vi "Window Title.vi"(0 "LV RT in":refnum<class "LV RT.lvclass">, 5 "VI Reference":refnum<vi>, 11 "error in (no error)":errorcluster) -> (4 "LV RT out":refnum<class "LV RT.lvclass">, 6 "Window Title":string, 15 "error out":errorcluster)   [LabVIEW 2016, in "LV RT.lvclass"]
uses:
  LV RT.lvclass
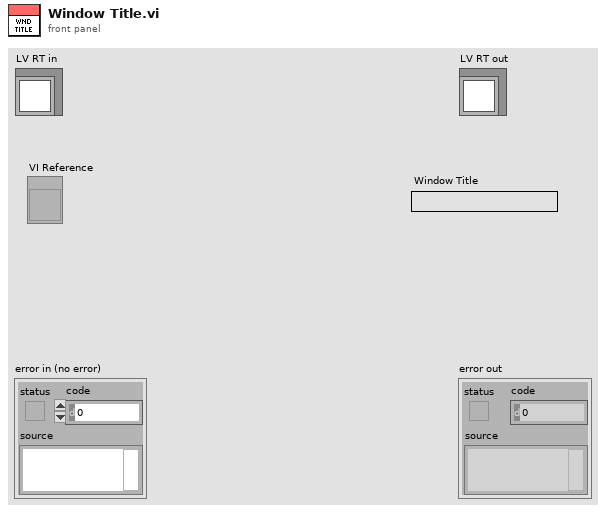
[diagram p1: front panel]
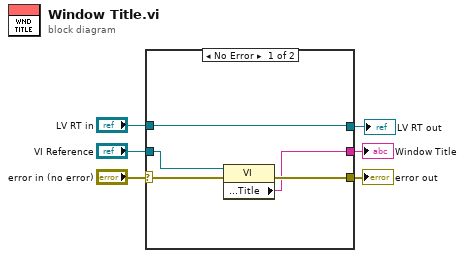
[diagram p0: block diagram]
diagram:
  n1 = case shown="No Error" "error in (no error)" {
    selector: "error in (no error)" -> [w11 w13]
    tunnel: [w9 w13] -> w5
    tunnel: "LV RT in" -> [w10 w12]
    tunnel: [w10 w12] -> w3
    tunnel: "VI Reference" -> [w8 _]
    tunnel: [w7 _] -> w1
    frame No Error {
      n2 = property class="VI"(reference=w8, error in=w11) -> (error out=w9:errorcluster, "Front Panel.Title"=w7:string)  [unwired: 1 out]
    }
    frame Error {
    }
  }
  "error out" <- w5
  "LV RT out" <- w3
  "Window Title" <- w1
